vi "niusrprios Initiate Stream.vi"(0 "niUsrpRio Session":T1={"FPGA Interface"=refnum, "RIO Interface Number"=0, "Data Clock Rate"=0, "FPGA Data Clock Rate"=0, "Global Settings Register Bus"=refnum, "Radio 0 Settings Register Bus"=refnum, "Radio 1 Settings Register Bus"=refnum, "Radio Settings Bus Semaphore"=refnum, "DB Queues"=[], "Characterization Data Valid?"=FALSE, "EEPROM Header"={"Checksum"=0, "Product Code"=0, "Hardware Current Version"=0, "Hardware Oldest Compatible Version"=0, "EEPROM Map Current Version"=0, "EEPROM Map Oldest Compatible Version"=0, "User Password"="", "Pointer to Factory Header"=0, "Pointer to User Header"=0, "Recommended Interval"=0, "Number of Reserved Bytes"=9, "Number of Daughterboards"=0, "Daughterboard IDs"=[], "Daughterboard Serial Numbers"=[]}, "Device Data Header"={"Checksum"=0, "Number of Channels"=0, "Number of Gain Settings"=[], "Pointer to Characterization Data"=[], "Number of Reserved Bytes"=27, "Number of Frequencies"=[]}, "EEPROM Characterization Header"={"Checksum"=0, "Date"=timestamp(0 s since 1904-01-01), "Temperature"=0.0, "Misc. Info"="", "Pointer to Device Data Header"=0, "Number of Reserved Bytes"=28}, "Characterization Data"=[], "FPGA Current Version"=0, "FPGA Oldest Compatible Version"=0, "Fixed Logic Current Version"=0, "Fixed Logic Oldest Compatible Version"=0, "FPGA Radio Settings Bus Current Version"=0, "FPGA Radio Settings Bus Oldest Compatible Version"=0, "FPGA Board Config Current Version"=0, "FPGA Board Config Oldest Compatible Version"=0, "Daughterboard Clock Rate"=0} {"Daughterboard Clock Rate" format="%#.3pHz"; "FPGA Data Clock Rate" format="%#.3pHz"; "Data Clock Rate" format="%#.3pHz"; "Characterization Data"."Frequencies [Hz]" format="%#_6p"; "EEPROM Characterization Header"."Pointer to Device Data Header" format="%x"; "EEPROM Characterization Header"."Checksum" format="%x"; "Device Data Header"."Pointer to Characterization Data" format="%x"; "Device Data Header"."Checksum" format="%x"; "EEPROM Header"."Pointer to User Header" format="%x"; "EEPROM Header"."Pointer to Factory Header" format="%x"; "EEPROM Header"."Product Code" format="%x"; "EEPROM Header"."Checksum" format="%x"}, 1 "scope":string(combo)="rx", 11 "error in":errorcluster) -> (4 "niUsrpRio Session (out)":T1={"FPGA Interface"=refnum, "RIO Interface Number"=0, "Data Clock Rate"=0, "FPGA Data Clock Rate"=0, "Global Settings Register Bus"=refnum, "Radio 0 Settings Register Bus"=refnum, "Radio 1 Settings Register Bus"=refnum, "Radio Settings Bus Semaphore"=refnum, "DB Queues"=[], "Characterization Data Valid?"=FALSE, "EEPROM Header"={"Checksum"=0, "Product Code"=0, "Hardware Current Version"=0, "Hardware Oldest Compatible Version"=0, "EEPROM Map Current Version"=0, "EEPROM Map Oldest Compatible Version"=0, "User Password"="", "Pointer to Factory Header"=0, "Pointer to User Header"=0, "Recommended Interval"=0, "Number of Reserved Bytes"=9, "Number of Daughterboards"=0, "Daughterboard IDs"=[], "Daughterboard Serial Numbers"=[]}, "Device Data Header"={"Checksum"=0, "Number of Channels"=0, "Number of Gain Settings"=[], "Pointer to Characterization Data"=[], "Number of Reserved Bytes"=27, "Number of Frequencies"=[]}, "EEPROM Characterization Header"={"Checksum"=0, "Date"=timestamp(0 s since 1904-01-01), "Temperature"=0.0, "Misc. Info"="", "Pointer to Device Data Header"=0, "Number of Reserved Bytes"=28}, "Characterization Data"=[], "FPGA Current Version"=0, "FPGA Oldest Compatible Version"=0, "Fixed Logic Current Version"=0, "Fixed Logic Oldest Compatible Version"=0, "FPGA Radio Settings Bus Current Version"=0, "FPGA Radio Settings Bus Oldest Compatible Version"=0, "FPGA Board Config Current Version"=0, "FPGA Board Config Oldest Compatible Version"=0, "Daughterboard Clock Rate"=0} {"Daughterboard Clock Rate" format="%#.3pHz"; "FPGA Data Clock Rate" format="%#.3pHz"; "Data Clock Rate" format="%#.3pHz"; "Characterization Data"."Frequencies [Hz]" format="%#_6p"; "EEPROM Characterization Header"."Pointer to Device Data Header" format="%x"; "EEPROM Characterization Header"."Checksum" format="%x"; "Device Data Header"."Pointer to Characterization Data" format="%x"; "Device Data Header"."Checksum" format="%x"; "EEPROM Header"."Pointer to User Header" format="%x"; "EEPROM Header"."Pointer to Factory Header" format="%x"; "EEPROM Header"."Product Code" format="%x"; "EEPROM Header"."Checksum" format="%x"}, 15 "error out":errorcluster)   [LabVIEW 2015]
doc: "Initiates the stream. This is required before you acquire/generate data with the Fetch Rx Data or Write Tx Data VIs. Initiation includes resetting the Rx/Tx streams and the DSP.\n\n<b>Multi-device usage:</b>\nInitiate the master device last, after initiating all the slave devices.\n\n<B>Input Parameters</B>\n\n<B>niUsrpRio Session</B> is the object created by the Open VI and used as the session handle for the USRP RIO design library.\n\n<B>scope</B> is the channel on which stream is to be initiated. The options are \"rx/RF 0\", \"rx/RF 1\", \"tx/RF 0\", and \"tx/RF 1\".\n\n<B>error in</B> describes error conditions that occur before this node runs. This input provides standard 'error in' functionality.\n\n<B>Output Parameters</B>\n\n<B>niUsrpRio Session (out)</B> is the niUsrpRio session used in all subsequent USRP RIO design library host VIs.\n\n<B>error out</B> contains error information. This output provides standard 'error out' functionality."
uses:
  <instrlib>/niUsrpRio/Config/v1/Host/Public/niUsrpRio Session.ctl
  <instrlib>/_niInstr/Register Bus/v0/Host/Public/Register Bus Session.ctl
  <instrlib>/_niInstr/Register Bus/v0/Host/Private/Session Data.ctl
  <instrlib>/niUsrpRio/Config/v1/Host/Private/DB Queue Reference.ctl
  <instrlib>/niUsrpRio/Config/v1/Host/Private/Daughterboard Data.ctl
  <instrlib>/niUsrpRio/Config/v1/Host/Private/ATR state data.ctl
  <instrlib>/niUsrpRio/Config/v1/Host/Private/Antenna Configuration.ctl
  <instrlib>/niUsrpRio/Config/v1/Host/Private/CPLD Power Mode.ctl
  <instrlib>/niUsrpRio/Config/v1/Host/Public/EEPROM Header.ctl
  <instrlib>/niUsrpRio/Config/v1/Host/Public/EEPROM Device Data Header.ctl
  <instrlib>/niUsrpRio/Config/v1/Host/Public/EEPROM Characterization Header.ctl
  <instrlib>/niUsrpRio/Config/v1/Host/Public/Characterization Data.ctl
  <instrlib>/niUsrpRio/Config/v1/Host/Public/IQ Imbalance.ctl
  niusrprios Streaming Xvcr FPGA Ref.ctl
  <vilib>/rvi/errors/niLvFpgaAdjustHostInterfaceError.vi
  <vilib>/Utility/error.llb/Error Cluster From Error Code.vi
  <vilib>/rvi/interface/nirviReadWriteControl/nirviReadWriteControl.xnode
  <vilib>/ErrorRing/Error Ring.xnode
  <vilib>/rvi/interface/Simulation/niFpgaSimulationCallBeginRW.vi
  NiFpgaLv.dll
  <instrlib>/niUsrpRio/Config/v1/Host/niUsrpRio Config v1 Host.lvlib
  <instrlib>/_niInstr/Register Bus/v0/Host/niInstr Register Bus v0 Host.lvlib
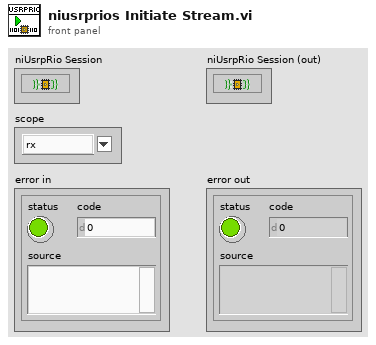
[diagram p1: front panel]
types:
  T1 = typedef "niUsrpRio Config v1 Host.lvlib/niUsrpRio Session.ctl" = cluster{"FPGA Interface":refnum<k20>, "RIO Interface Number":u32, "Data Clock Rate":u32, "FPGA Data Clock Rate":u32, "Global Settings Register Bus":T2, "Radio 0 Settings Register Bus":T2, "Radio 1 Settings Register Bus":T2, "Radio Settings Bus Semaphore":T3, "DB Queues":T4[], "Characterization Data Valid?":bool, "EEPROM Header":T5, "Device Data Header":T6, "EEPROM Characterization Header":T7, "Characterization Data":T8[], "FPGA Current Version":u32, "FPGA Oldest Compatible Version":u32, "Fixed Logic Current Version":u32, "Fixed Logic Oldest Compatible Version":u32, "FPGA Radio Settings Bus Current Version":u32, "FPGA Radio Settings Bus Oldest Compatible Version":u32, "FPGA Board Config Current Version":u32, "FPGA Board Config Oldest Compatible Version":u32, "Daughterboard Clock Rate":u32}
  T2 = typedef "niInstr Register Bus v0 Host.lvlib/Register Bus Session.ctl" = refnum<queue>
  T3 = typedef "Semaphore RefNum" = refnum<k1>
  T4 = typedef "niUsrpRio Config v1 Host.lvlib/DB Queue Reference.ctl" = refnum<queue>
  T5 = typedef "niUsrpRio Config v1 Host.lvlib/EEPROM Header.ctl" = cluster{"Checksum":u32, "Product Code":u16, "Hardware Current Version":u16, "Hardware Oldest Compatible Version":u16, "EEPROM Map Current Version":u16, "EEPROM Map Oldest Compatible Version":u16, "User Password":string, "Pointer to Factory Header":u32, "Pointer to User Header":u32, "Recommended Interval":u16, "Number of Reserved Bytes":i32, "Number of Daughterboards":u8, "Daughterboard IDs":u16[], "Daughterboard Serial Numbers":string[]}
  T6 = typedef "niUsrpRio Config v1 Host.lvlib/EEPROM Device Data Header.ctl" = cluster{"Checksum":u32, "Number of Channels":u8, "Number of Gain Settings":u16[], "Pointer to Characterization Data":u32[], "Number of Reserved Bytes":i32, "Number of Frequencies":u16[]}
  T7 = typedef "niUsrpRio Config v1 Host.lvlib/EEPROM Characterization Header.ctl" = cluster{"Checksum":u32, "Date":timestamp, "Temperature":sgl, "Misc. Info":string, "Pointer to Device Data Header":u32, "Number of Reserved Bytes":i32}
  T8 = typedef "niUsrpRio Config v1 Host.lvlib/Characterization Data.ctl" = cluster{"Gains[dB]":dbl[], "Frequencies [Hz]":dbl[], "IQ Imbalance Table":T9[], "Measured Gains[dB]":dbl[][]}
  T9 = typedef "niUsrpRio Config v1 Host.lvlib/IQ Imbalance.ctl" = cluster{"Gain Imbalance [linear]":dbl, "Phase Imbalance [radians]":dbl, "Offset":cdb}
  T10 = typedef "niusrprios Streaming Xvcr FPGA Ref.ctl" = refnum<k20>
  T11 = typedef "niUsrpRio Config v1 Host.lvlib/Device Subfunction.ctl" = enum16{"rx", "tx", "all"}
  T12 = typedef "niUsrpRio Config v1 Host.lvlib/RF Channel.ctl" = enum16{"0", "1", "All"}
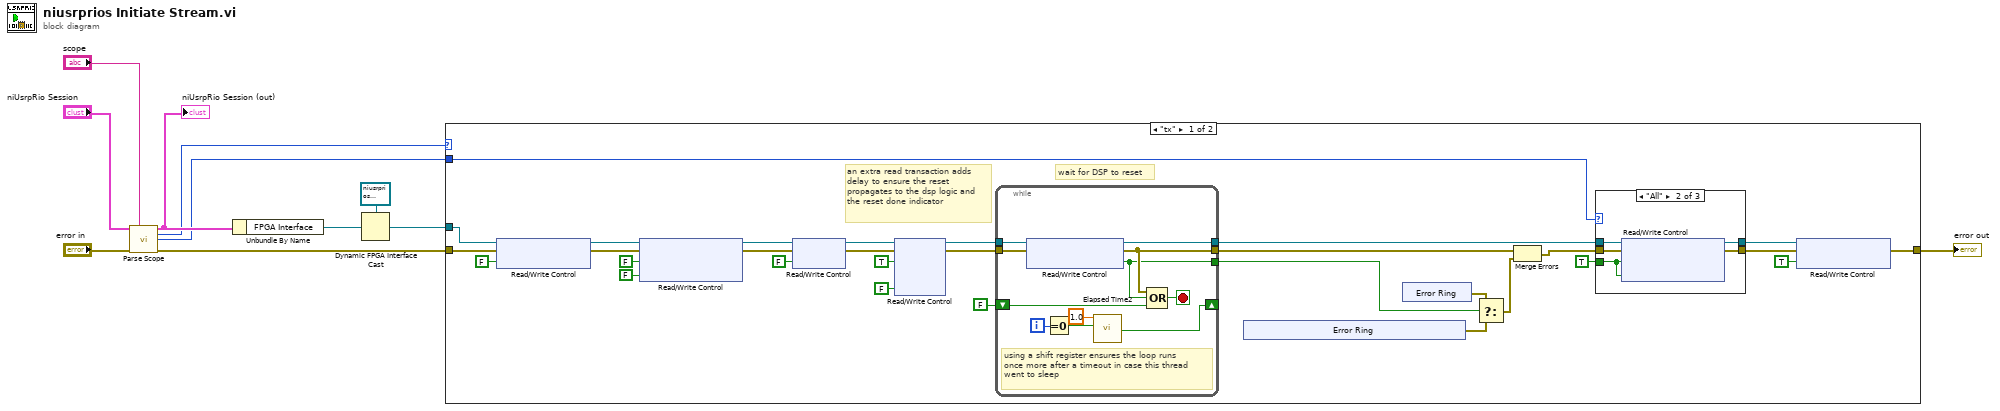
[diagram p0: block diagram]
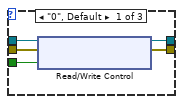
[diagram p2: hidden frame]
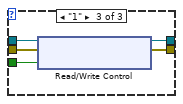
[diagram p3: hidden frame]
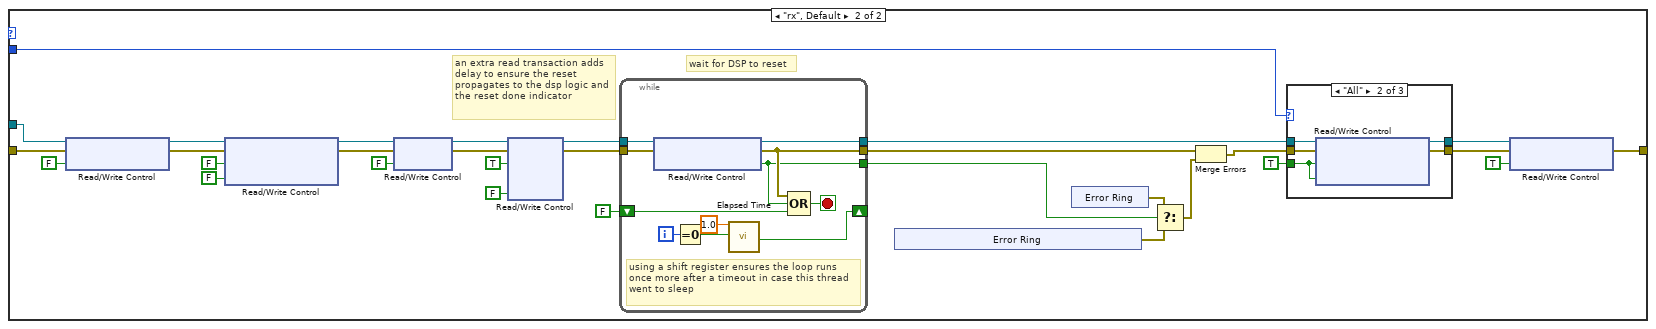
[diagram p4: hidden frame]
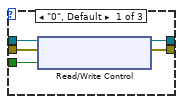
[diagram p5: hidden frame]
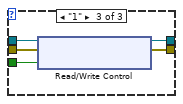
[diagram p6: hidden frame]
diagram:
  n1 = call <instrlib>:"Parse Scope.vi"("niUsrpRio Session"="niUsrpRio Session", "scope"="scope", "error in"="error in") -> ("niUsrpRio Session (out)"=w11:T1, "Device Subfunction"=w8:T11, "Device Subfunction Channel"=w7:T12, "error out"=w6:errorcluster)  [unwired: 4 in, 5 out]
  "niUsrpRio Session (out)" <- w11
  n2 = Unbundle By Name(w11) -> ("FPGA Interface"=w4:refnum<k20>)
  n3 = Dynamic FPGA Interface Cast(Session In=T10 refnum ("Type"), Type=w4) -> (Session Out=w3:T10)
  n4 = case shown="\"tx\"" w8 {
    tunnel: w3 -> [w25 w85]
    tunnel: [w26 w86] -> w2
    tunnel: w6 -> [w32 w92]
    tunnel: w7 -> [w33 w93]
    frame "tx" {
      # "an extra read transaction adds delay to ensure the reset propagates to the dsp logic and the reset done indicator"
      # "wait for DSP to reset"
      n5 = xnode "Read/Write Control"("FPGA VI Reference In"=w25, "error in"=w32, "tx.trigger enable"=FALSE) -> ("FPGA VI Reference Out"=w30:T10, "error out"=w31:errorcluster)
      n6 = xnode "Read/Write Control"("FPGA VI Reference In"=w30, "error in"=w31, "tx 0.stream enable"=FALSE, "tx 1.stream enable"=FALSE) -> ("FPGA VI Reference Out"=w36:T10, "error out"=w37:errorcluster)
      n7 = xnode "Read/Write Control"("FPGA VI Reference In"=w36, "error in"=w37, "tx.abort"=FALSE) -> ("FPGA VI Reference Out"=w17:T10, "error out"=w16:errorcluster)
      n8 = xnode "Read/Write Control"("FPGA VI Reference In"=w17, "error in"=w16, "tx.reset"=TRUE, "tx.reset"=FALSE) -> ("FPGA VI Reference Out"=w13:T10, "error out"=w14:errorcluster)  [unwired: 1 out]
      n9 = while {
        tunnel: [w69] -> w20
        tunnel: [w68] -> w19
        shift-right: [w66] -> _
        shift-left: FALSE ("Time has Elapsed") -> [w67]
        tunnel: [w65] -> w21
        tunnel: w14 -> [w64]
        tunnel: w13 -> [w63]
        i -> [w72]
        stop <- w70 stop-if-true
        # "using a shift register ensures the loop runs once more after a timeout in case this thread went to sleep"
        n10 = xnode "Read/Write Control"("FPGA VI Reference In"=w63, "error in"=w64) -> ("FPGA VI Reference Out"=w68:T10, "error out"=w69:errorcluster, "tx.dsp reset done"=w65:bool)
        n11 = Equal To 0?(x=w72) -> (x = 0?=w73:bool)
        n12 = call "Elapsed Time2"("Time Target (s)"=1.0, "Reset"=w73) -> ("Time has Elapsed"=w66:bool)  [unwired: 10 in, 7 out]
        n13 = Compound Arithmetic op=OR(w69, w65, w67) -> (w70:bool)
      }
      n14 = xnode "Error Ring"() -> ("error out"=w38:errorcluster)
      n15 = xnode "Error Ring"() -> ("error out"=w39:errorcluster)
      n16 = Select(t=w39, s=w21, f=w38) -> (s? t:f=w40:errorcluster)
      n17 = Merge Errors(w20, w40) -> (w34:errorcluster)
      n18 = case shown="\"All\"" w33 {
        tunnel: w34 -> [w46 w51 w56]
        tunnel: w19 -> [w45 w50 w52]
        tunnel: [w44 w49 w54] -> w27
        tunnel: [w43 w48 w55] -> w28
        tunnel: TRUE ("tx.stream enabled") -> [w42 w47 w53]
        frame "0", Default {
          n19 = xnode "Read/Write Control"("FPGA VI Reference In"=w45, "error in"=w46, "tx 0.stream enable"=w42) -> ("FPGA VI Reference Out"=w43:T10, "error out"=w44:errorcluster)
        }
        frame "All" {
          n20 = xnode "Read/Write Control"("FPGA VI Reference In"=w50, "error in"=w51, "tx 0.stream enable"=w47, "tx 1.stream enable"=w47) -> ("FPGA VI Reference Out"=w48:T10, "error out"=w49:errorcluster)
        }
        frame "1" {
          n21 = xnode "Read/Write Control"("FPGA VI Reference In"=w52, "error in"=w56, "tx 1.stream enable"=w53) -> ("FPGA VI Reference Out"=w55:T10, "error out"=w54:errorcluster)
        }
      }
      n22 = xnode "Read/Write Control"("FPGA VI Reference In"=w28, "error in"=w27, "tx.trigger enable"=TRUE ("tx.enable trigger")) -> ("error out"=w26:errorcluster)  [unwired: 1 out]
    }
    frame "rx", Default {
      # "an extra read transaction adds delay to ensure the reset propagates to the dsp logic and the reset done indicator"
      # "wait for DSP to reset"
      n23 = xnode "Read/Write Control"("FPGA VI Reference In"=w85, "error in"=w92, "rx.trigger enable"=FALSE ("tx.trigger enable")) -> ("FPGA VI Reference Out"=w90:T10, "error out"=w91:errorcluster)
      n24 = xnode "Read/Write Control"("FPGA VI Reference In"=w90, "error in"=w91, "rx 0.stream enable"=FALSE ("tx 0.stream enable"), "rx 1.stream enable"=FALSE ("tx 1.stream enable")) -> ("FPGA VI Reference Out"=w96:T10, "error out"=w97:errorcluster)
      n25 = xnode "Read/Write Control"("FPGA VI Reference In"=w96, "error in"=w97, "rx.abort"=FALSE ("tx.abort")) -> ("FPGA VI Reference Out"=w101:T10, "error out"=w102:errorcluster)
      n26 = xnode "Read/Write Control"("FPGA VI Reference In"=w101, "error in"=w102, "rx.reset"=TRUE ("tx.reset"), "rx.reset"=FALSE ("tx.reset")) -> ("FPGA VI Reference Out"=w74:T10, "error out"=w75:errorcluster)  [unwired: 1 out]
      n27 = while {
        tunnel: w74 -> [w135]
        tunnel: w75 -> [w134]
        tunnel: [w129] -> w80
        tunnel: [w128] -> w79
        shift-right: [w126] -> _
        shift-left: FALSE ("Time has Elapsed") -> [w127]
        tunnel: [w125] -> w81
        i -> [w132]
        stop <- w130 stop-if-true
        # "using a shift register ensures the loop runs once more after a timeout in case this thread went to sleep"
        n28 = xnode "Read/Write Control"("FPGA VI Reference In"=w135, "error in"=w134) -> ("FPGA VI Reference Out"=w128:T10, "error out"=w129:errorcluster, "rx.dsp reset done"=w125:bool)
        n29 = Equal To 0?(x=w132) -> (x = 0?=w133:bool)
        n30 = call "Elapsed Time"("Time Target (s)"=1.0, "Reset"=w133) -> ("Time has Elapsed"=w126:bool)  [unwired: 10 in, 7 out]
        n31 = Compound Arithmetic op=OR(w129, w125, w127) -> (w130:bool)
      }
      n32 = xnode "Error Ring"() -> ("error out"=w98:errorcluster)
      n33 = xnode "Error Ring"() -> ("error out"=w99:errorcluster)
      n34 = Select(t=w99, s=w81, f=w98) -> (s? t:f=w100:errorcluster)
      n35 = Merge Errors(w80, w100) -> (w94:errorcluster)
      n36 = case shown="\"All\"" w93 {
        tunnel: w94 -> [w108 w113 w118]
        tunnel: w79 -> [w107 w112 w114]
        tunnel: [w106 w111 w116] -> w87
        tunnel: [w105 w110 w117] -> w88
        tunnel: TRUE ("tx.stream enabled") -> [w104 w109 w115]
        frame "0", Default {
          n37 = xnode "Read/Write Control"("FPGA VI Reference In"=w107, "error in"=w108, "rx 0.stream enable"=w104) -> ("FPGA VI Reference Out"=w105:T10, "error out"=w106:errorcluster)
        }
        frame "All" {
          n38 = xnode "Read/Write Control"("FPGA VI Reference In"=w112, "error in"=w113, "rx 0.stream enable"=w109, "rx 1.stream enable"=w109) -> ("FPGA VI Reference Out"=w110:T10, "error out"=w111:errorcluster)
        }
        frame "1" {
          n39 = xnode "Read/Write Control"("FPGA VI Reference In"=w114, "error in"=w118, "rx 1.stream enable"=w115) -> ("FPGA VI Reference Out"=w117:T10, "error out"=w116:errorcluster)
        }
      }
      n40 = xnode "Read/Write Control"("FPGA VI Reference In"=w88, "error in"=w87, "rx.trigger enable"=TRUE ("tx.enable trigger")) -> ("error out"=w86:errorcluster)  [unwired: 1 out]
    }
  }
  "error out" <- w2
